vi "GT Get Home Status.vi"(8 "error in (no error)":errorcluster caption="错误输入（无错误）", 9 "pHomeStatus":T1, 10 "axis":i16, 11 "cardNum":i16) -> (0 "error out":errorcluster caption="错误输出", 1 "pHomeStatus out":T1, 3 "function return":i16)   [LabVIEW 2014, in "gts.lvlib"]
doc: "GT_API GT_GetHomeStatus(short cardNum,short axis,THomeStatus *pHomeStatus);"
uses:
  gts.lvlib
  gts.dll
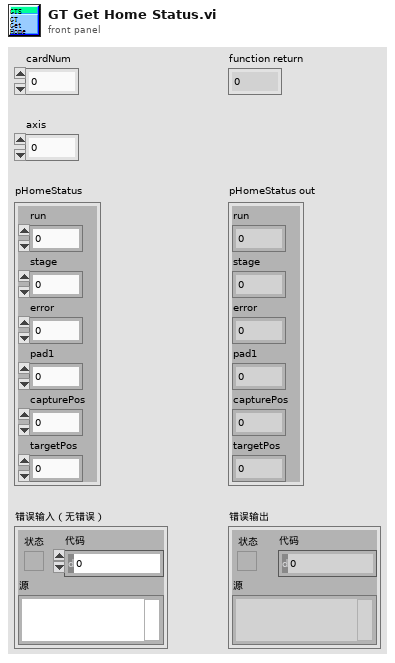
[diagram p1: front panel]
types:
  T1 = cluster{"run":i16, "stage":i16, "error":i16, "pad1":i16, "capturePos":i32, "targetPos":i32}
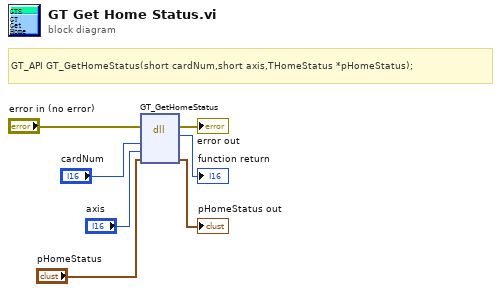
[diagram p0: block diagram]
diagram:
  # "GT_API GT_GetHomeStatus(short cardNum,short axis,THomeStatus *pHomeStatus);"
  n1 = dll-call lib="PTH2>abs F.多卡库-控制卡基本运动例程(labview)gts.*" fn="GT_GetHomeStatus"(error in="error in (no error)", "cardNum"="cardNum", "axis"="axis", "pHomeStatus"="pHomeStatus") -> (error out=→"error out":errorcluster, →"function return":i16, "pHomeStatus"=→"pHomeStatus out":T1)  [unwired: 4 in, 1 out]
